vi "Locate SCM Breakdown Lib.vi"(0 "Signals":dbl[][](array[numeric]), 5 "Sampling Rate (S/s)":i32, 7 "Offset (µs)":dbl format="%#_13g", 9 "Duration (µs)":dbl format="%#_13g", 11 "error in (no error)":errorcluster, 13 "Microphone Coordinates (cm, rad)":cluster{"r":dbl, "theta":dbl}[](array[cluster])) -> (4 "Coordinates (cm, rad, cm)":cluster{"r":sgl, "theta":sgl, "z":sgl}[](array[cluster]), 15 "error out":errorcluster)   [LabVIEW 2013]
uses:
  <userlib>/liblocalize/liblocalize.lvlib
panel:
  out "Window":i32[](array[numeric])
  out "Downstream Signals":dbl[][](graph)
  out "Upstream Signals":dbl[][](graph)
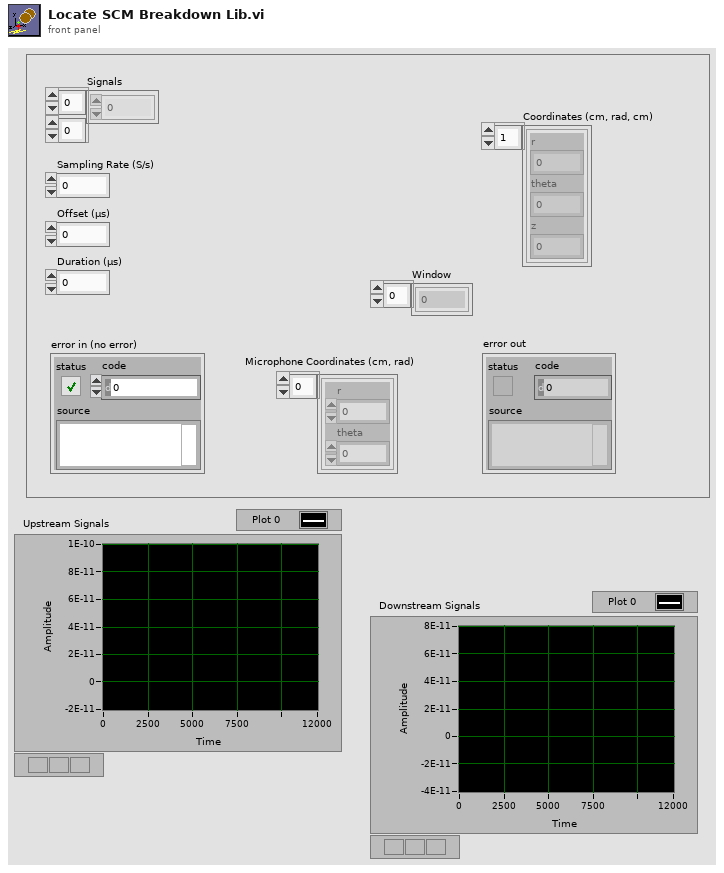
[diagram p1: front panel]
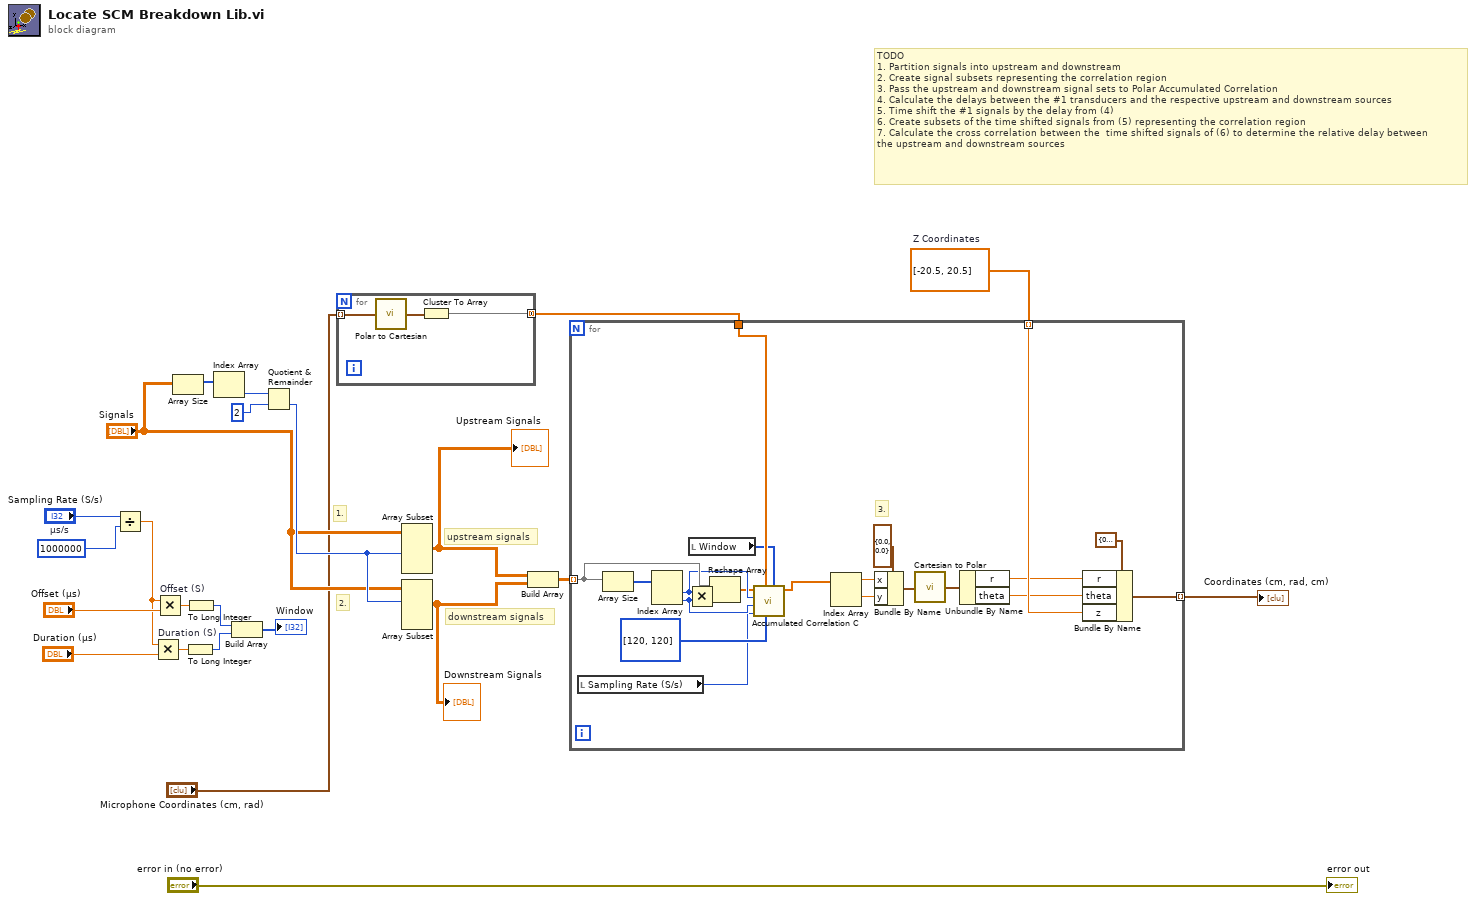
[diagram p0: block diagram]
diagram:
  w19 = dbl[] [-20.5, 20.5]  # Z Coordinates
  w11 = 1000000  # µs/s
  # "2."
  # "1."
  # "downstream signals"
  # "upstream signals"
  # "TODO\n1. Partition signals into upstream and downstream\n2. Create signal subsets representing the correlation region\n3. Pass the upstream and downstream signal sets to Polar Accumulated Correlation\n4. Calculate the delays between the #1 transducers and the respective upstream and downstream sources\n5. Time shift the #1 signals by the delay from (4)\n6. Create subsets of the time shifted signals from (5) representing the correlation region\n7. Calculate the cross correlation between the  time shifted signals of (6) to determine the relative delay between\nthe upstream and downstream sources"
  n1 = Divide(x="Sampling Rate (S/s)", y=w11) -> (x/y=w20:dbl)
  n2 = Multiply "Duration (S)"(x=w20, y="Duration (µs)") -> (x*y=w4:dbl)
  n3 = Multiply "Offset (S)"(x=w20, y="Offset (µs)") -> (x*y=w5:dbl)
  n4 = Array Size(array="Signals") -> (size(s)=w16:i32[])
  n5 = To Long Integer(number=w4) -> (32bit integer=w2:i32)
  n6 = To Long Integer(number=w5) -> (32bit integer=w3:i32)
  n7 = Index Array(array=w16) -> (element=w15:i32)  [unwired: 1 in]
  n8 = Build Array(w3, w2) -> (→"Window":i32[])
  n9 = Quotient & Remainder(x=w15, y=2) -> (floor(x/y)=w13:i32)  [unwired: 1 out]
  n10 = for {
    tunnel: "Microphone Coordinates (cm, rad)" -> [w26] mode=indexing
    tunnel: [w24] -> w6 mode=concatenating
    n11 = call "Polar to Cartesian.vi"("Polar\nCoordinates"=w26) -> ("Cartesian\nCoordinates"=w25:cluster{"x":dbl, "y":dbl})  [unwired: 4 in]
    n12 = Cluster To Array(cluster=w25) -> (array=w24:dbl[])
  }
  n13 = Array Subset(array="Signals", length (row)=w13) -> (w9:dbl[][])  [unwired: 3 in]
  "Upstream Signals" <- w9
  n14 = Array Subset(array="Signals", index (row)=w13) -> (w8:dbl[][])  [unwired: 3 in]
  "Downstream Signals" <- w8
  n15 = Build Array(w9, w8) -> (w23:dbl[][][])
  n16 = for {
    tunnel: w23 -> [w42] mode=indexing
    tunnel: w19 -> [w47] mode=indexing
    tunnel: [w46] -> w18 mode=indexing
    tunnel: w6 -> [w30]
    # "3."
    n17 = local read "Sampling Rate (S/s)"() -> (w28:i32)
    n18 = Array Size(array=w42) -> (size(s)=w41:i32[])
    n19 = Index Array(array=w41) -> (element #1=w34:i32, element #2=w32:i32)  [unwired: 2 in]
    n20 = Multiply(x=w34, y=w32) -> (x*y=w40:i32)
    n21 = local read "Window"() -> (w27:i32[])
    n22 = Reshape Array(w42, w40) -> (w33:dbl[])
    n23 = call <userlib>:"Accumulated Correlation C.vi"("window"=w27, "resolution"=u64[] [120, 120], "mic_coords"=w30, "sampling_rate"=w28, "signal_length"=w32, "num_channels"=w34, "signals"=w33) -> ("coordinates"=w29:dbl[])  [unwired: 4 in]
    n24 = Index Array(array=w29) -> (element #1=w38:dbl, element #2=w37:dbl)  [unwired: 2 in]
    n25 = Bundle By Name(cluster=cluster{"x":dbl, "y":dbl} {"x"=0.0, "y"=0.0} ("input cluster"), "x"=w38, "y"=w37) -> (w36:cluster{"x":dbl, "y":dbl})
    n26 = call "Cartesian to Polar.vi"("Cartesian\nCoordinates"=w36) -> ("Polar\nCoordinates"=w35:cluster{"r":dbl, "theta":dbl})  [unwired: 4 in]
    n27 = Unbundle By Name(w35) -> ("r"=w45:dbl, "theta"=w44:dbl)
    n28 = Bundle By Name(cluster=cluster{"r":sgl, "theta":sgl, "z":sgl} {"r"=0.0, "theta"=0.0, "z"=0.0} ("Coordinates (m)"), "r"=w45, "theta"=w44, "z"=w47) -> (w46:cluster{"r":sgl, "theta":sgl, "z":sgl})
  }
  "Coordinates (cm, rad, cm)" <- w18
  "error out" <- "error in (no error)"
